vi "MovePosition.vi"(10 "Direction":T1, 11 "PlayerPosition":T2) -> (3 "NewPlayerPosition":T2)   [LabVIEW 2015, in "TronVIEWGameUtilities.lvlib"]
uses:
  TronVIEWGameUtilities.lvlib
  TronviewGame/Board/Position.ctl
  TronVIEWBotAPI/MovementDirection.ctl
  TronviewGame/Board/Board.lvclass
  TronVIEWBotAPI/TronVIEWBotAPI.lvlib
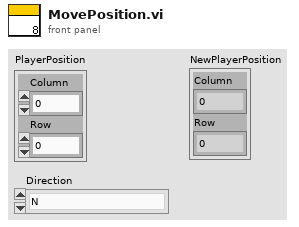
[diagram p1: front panel]
types:
  T1 = typedef "TronVIEWBotAPI.lvlib/MovementDirection.ctl" = enum16{"N", "S", "W", "E"}
  T2 = typedef "TronviewGame.lvlib/Board.lvclass/Position.ctl" = cluster{"Column":i32, "Row":i32}
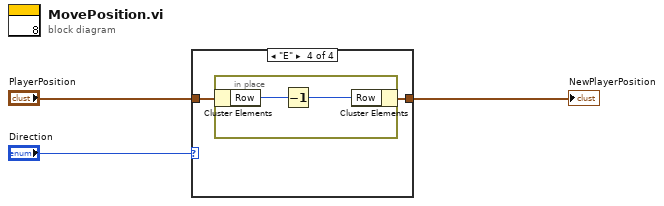
[diagram p0: block diagram]
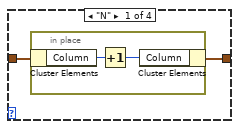
[diagram p2: hidden frame]
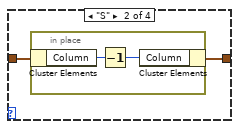
[diagram p3: hidden frame]
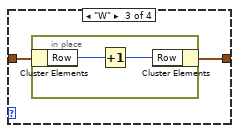
[diagram p4: hidden frame]
diagram:
  n1 = case shown="\"E\"" "Direction" {
    tunnel: "PlayerPosition" -> [w5 w9 w13 w17]
    tunnel: [w4 w8 w12 w16] -> w2
    frame "N" {
      n2 = in-place {
        n3 = in-place-cluster #1(w5) -> ("Column"=w7:i32)
        n4 = Increment(x=w7) -> (x+1=w6:i32)
        n5 = in-place-cluster #1("Column"=w6) -> (w4:T2)
      }
    }
    frame "S" {
      n6 = in-place {
        n7 = in-place-cluster #2(w9) -> ("Column"=w11:i32)
        n8 = Decrement(x=w11) -> (x-1=w10:i32)
        n9 = in-place-cluster #2("Column"=w10) -> (w8:T2)
      }
    }
    frame "W" {
      n10 = in-place {
        n11 = in-place-cluster #3(w13) -> ("Row"=w15:i32)
        n12 = Increment(x=w15) -> (x+1=w14:i32)
        n13 = in-place-cluster #3("Row"=w14) -> (w12:T2)
      }
    }
    frame "E" {
      n14 = in-place {
        n15 = in-place-cluster #4(w17) -> ("Row"=w19:i32)
        n16 = Decrement(x=w19) -> (x-1=w18:i32)
        n17 = in-place-cluster #4("Row"=w18) -> (w16:T2)
      }
    }
  }
  "NewPlayerPosition" <- w2
